vi "getSetting.vi"(7 "Array Parameter List":string[](array[string])=["izn3", "icomp"], 8 "error in (no error)":errorcluster, 9 "Parameter":string="estimator_strategy", 10 "Path":path=path "/home/ttsai/Documents/stash/ts_tcs_ofc/configData/pinv.esti", 11 "MatOper in":refnum<class "MatOper.lvclass">) -> (0 "error out":errorcluster, 2 "Value":string, 3 "MatOper out":refnum<class "MatOper.lvclass">)   [LabVIEW 2016, in "OfcFunc.lvlib" / "MatOper.lvclass"]
doc: "This vi is to read the configuration file based on the Parameter. This output can is the string. Array Parameter List defines the output with the array-like string data."
uses:
  MatOper.lvclass
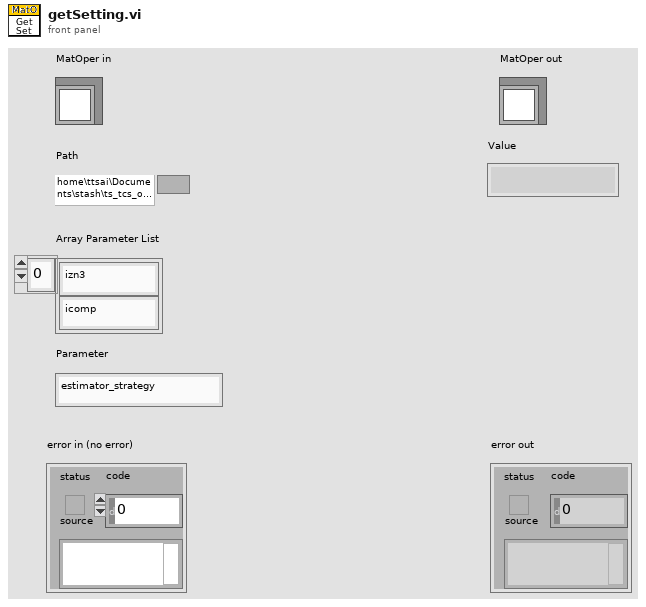
[diagram p1: front panel]
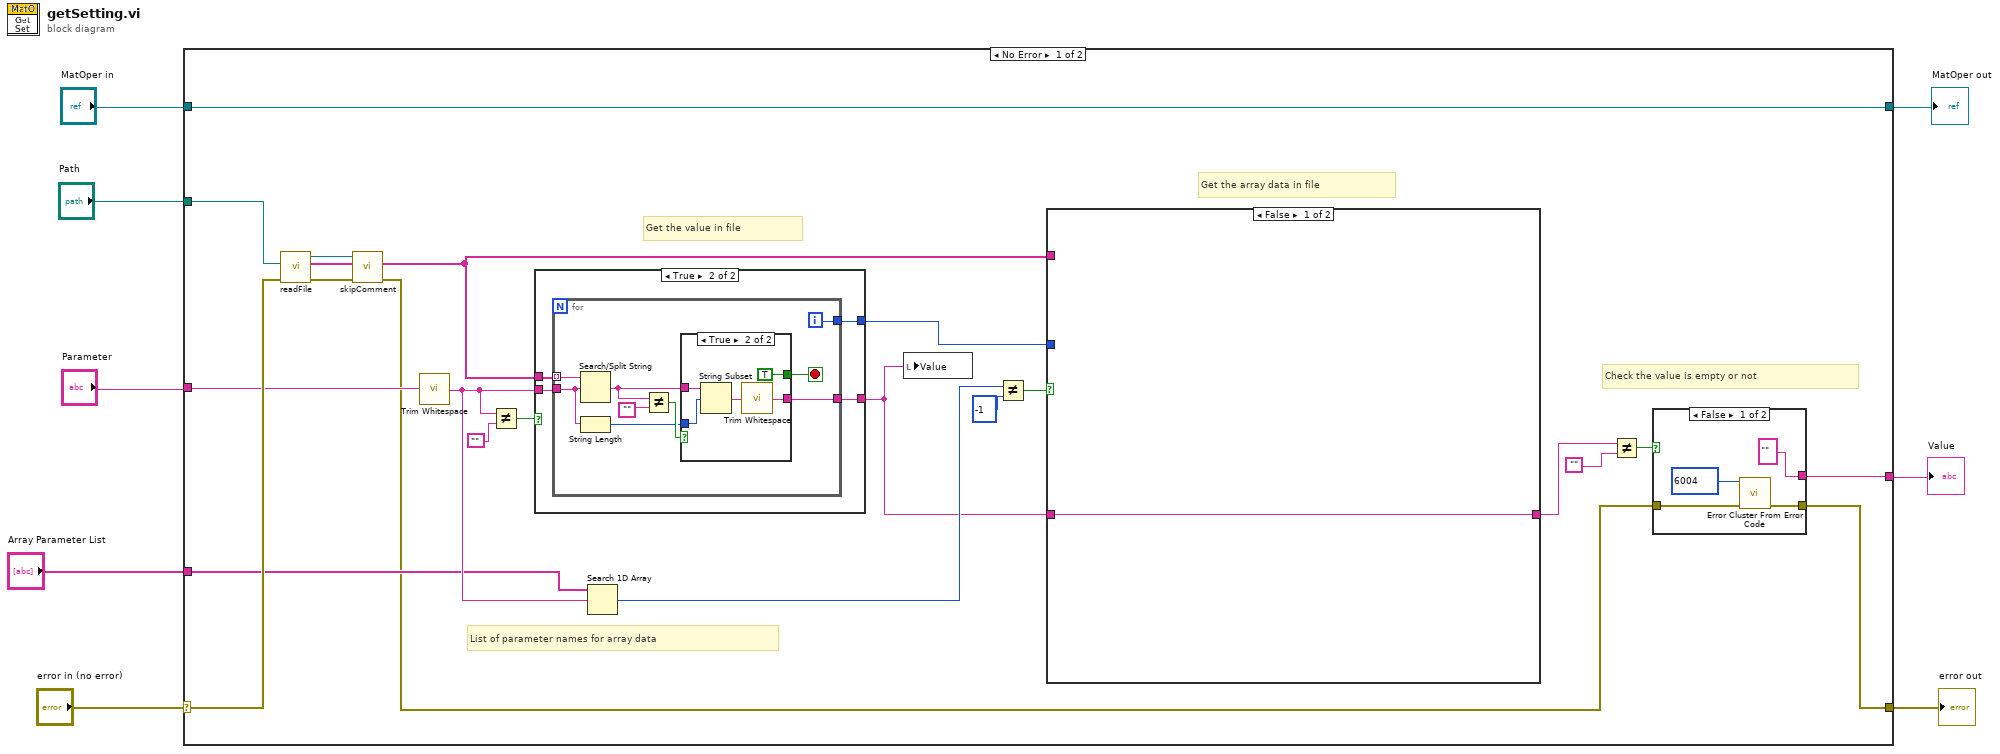
[diagram p0: block diagram]
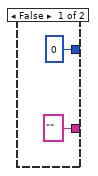
[diagram p2: hidden frame]
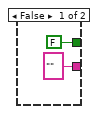
[diagram p3: hidden frame]
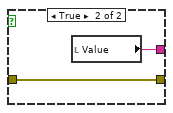
[diagram p4: hidden frame]
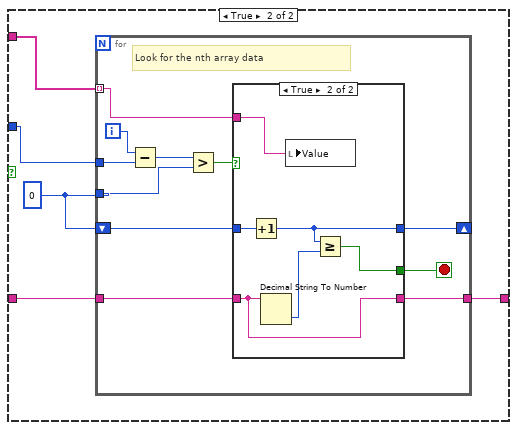
[diagram p5: hidden frame]
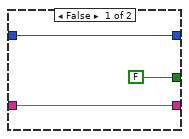
[diagram p6: hidden frame]
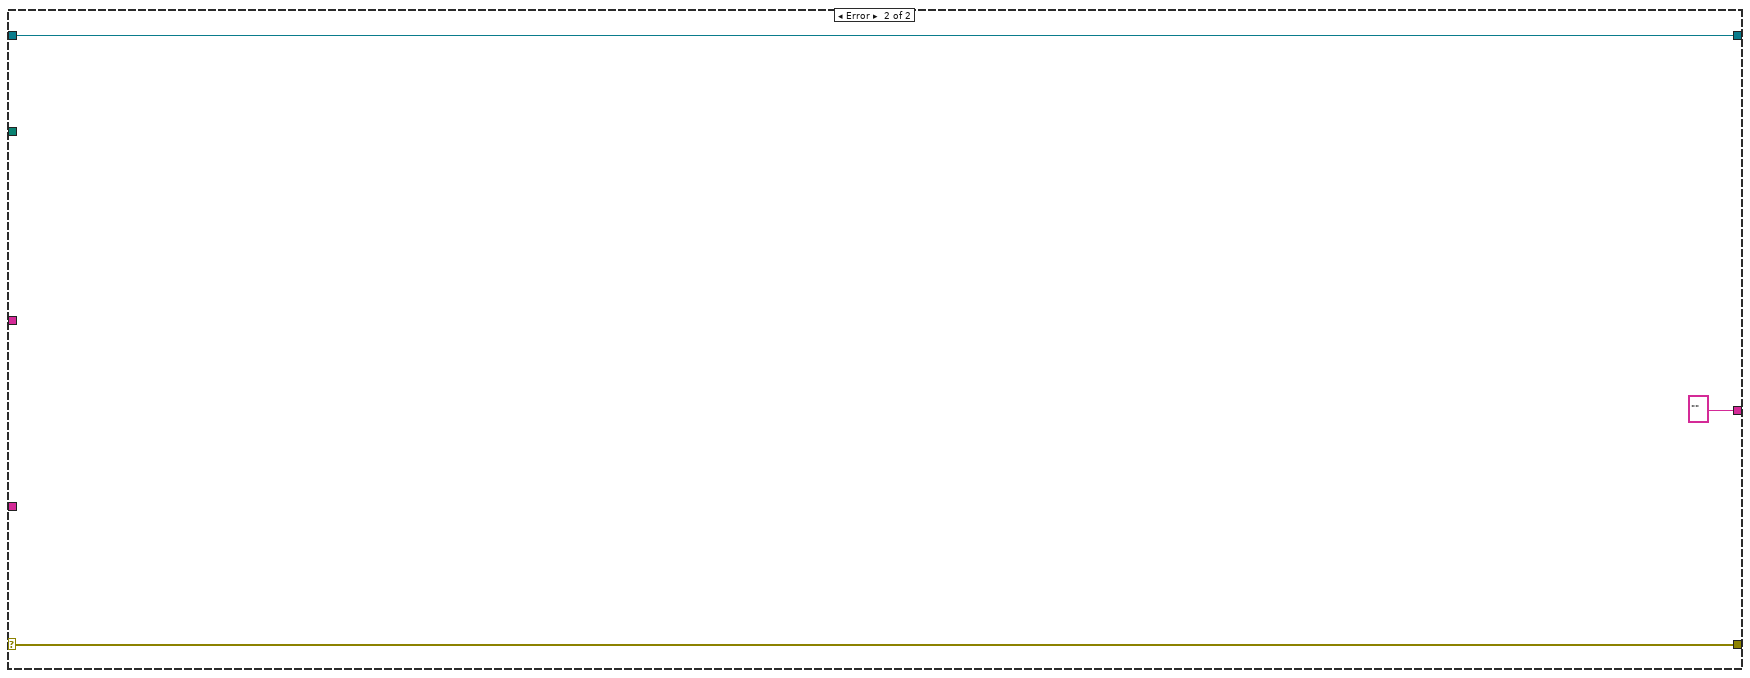
[diagram p7: hidden frame]
diagram:
  n1 = case shown="No Error" "error in (no error)" {
    selector: "error in (no error)" -> [w18 w88]
    tunnel: [w10 w88] -> w7
    tunnel: [w31 w87] -> w5
    tunnel: "MatOper in" -> [w31 w87]
    tunnel: "Path" -> [w17 _]
    tunnel: "Parameter" -> [w16 _]
    tunnel: "Array Parameter List" -> [w15 _]
    tunnel: [w9 "" ("Value")] -> w1
    frame No Error {
      # "Check the value is empty or not"
      # "List of parameter names for array data"
      # "Get the array data in file"
      # "Get the value in file"
      n2 = call "readFile.vi"("error in (no error)"=w18, "Path"=w17) -> ("error out"=w13:errorcluster, "Array"=w26:string[], "MatOper out"=w14:refnum<class "MatOper.lvclass">)  [unwired: 7 in]
      n3 = call "skipComment.vi"("error in (no error)"=w13, "Content"=w26, "MatOper in"=w14) -> ("error out"=w12:errorcluster, "Modified Content"=w25:string[])  [unwired: 6 in, 1 out]
      n4 = call <vilib>:"Trim Whitespace.vi"("string"=w16) -> ("trimmed string"=w20:string)  [unwired: 1 in]
      n5 = Not Equal?(x=w20, y="") -> (x != y?=w19:bool)
      n6 = case shown="True" w19 {
        tunnel: [0 w37] -> w27
        tunnel: ["" ("trimmed string") w36] -> w11
        tunnel: w25 -> [_ w35]
        tunnel: w20 -> [_ w34]
        frame False {
        }
        frame True {
          n7 = for {
            tunnel: w35 -> [w39] mode=indexing
            tunnel: w34 -> [w42]
            tunnel: [w41] -> w36
            tunnel: [w40] -> w37
            i -> [w40]
            stop <- w45 stop-if-true
            n8 = Search/Split String(string=w39, search string/char (-)=w42) -> (match + rest of string=w44:string)  [unwired: 1 in, 2 out]
            n9 = String Length(string=w42) -> (length=w43:i32)
            n10 = Not Equal?(x=w44, y="") -> (x != y?=w46:bool)
            n11 = case shown="True" w46 {
              tunnel: [FALSE TRUE] -> w45
              tunnel: w44 -> [_ w52]
              tunnel: ["" w49] -> w41
              tunnel: w43 -> [_ w51]
              frame False {
              }
              frame True {
                n12 = String Subset(string=w52, offset (0)=w51) -> (substring=w50:string)  [unwired: 1 in]
                n13 = call <vilib>:"Trim Whitespace.vi"("string"=w50) -> ("trimmed string"=w49:string)  [unwired: 1 in]
              }
            }
          }
        }
      }
      n14 = Search 1D Array(1D array=w15, element=w20) -> (index of element=w29:i32)  [unwired: 1 in]
      n15 = local write "Value"(w11) -> ()
      n16 = Not Equal?(x=w29, y=-1) -> (x != y?=w30:bool)
      n17 = case shown="False" w30 {
        tunnel: w27 -> [_ w65]
        tunnel: w25 -> [_ w64]
        tunnel: w11 -> [w60 w63]
        tunnel: [w60 w61] -> w22
        frame False {
        }
        frame True {
          w62 = 0 ("y")
          n18 = for {
            tunnel: w65 -> [w72]
            tunnel: w64 -> [w75] mode=indexing
            shift-right: [w68] -> _
            shift-left: w62 -> [w69]
            tunnel: w62 -> [w70]
            tunnel: w63 -> [w67]
            tunnel: [w66] -> w61
            i -> [w73]
            stop <- w71 stop-if-true
            # "Look for the nth array data"
            n19 = Subtract(x=w73, y=w72) -> (x-y=w74:i32)
            n20 = Greater?(x=w74, y=w70) -> (0:w76:bool)
            n21 = case shown="True" w76 {
              tunnel: w75 -> [_ w83]
              tunnel: [FALSE w84] -> w71
              tunnel: w69 -> [w78 w82]
              tunnel: [w78 w81] -> w68
              tunnel: w67 -> [w77 w80]
              tunnel: [w77 w80] -> w66
              frame False {
              }
              frame True {
                n22 = Increment(x=w82) -> (x+1=w81:i32)
                n23 = Decimal String To Number(string=w80) -> (number=w85:i32)  [unwired: 2 in, 1 out]
                n24 = local write "Value"(w83) -> ()
                n25 = Greater Or Equal?(x=w81, y=w85) -> (x >= y?=w84:bool)
              }
            }
          }
        }
      }
      n26 = Not Equal?(x=w22, y="") -> (x != y?=w24:bool)
      n27 = case shown="False" w24 {
        tunnel: w12 -> [w56 w59]
        tunnel: [w55 w59] -> w10
        tunnel: ["" ("Value") w58] -> w9
        frame False {
          n28 = call <vilib>:"Error Cluster From Error Code.vi"("error in (no error)"=w56, "error code (0)"=6004 ("code")) -> ("error out"=w55:errorcluster)  [unwired: 7 in]
        }
        frame True {
          n29 = local read "Value"() -> (w58:string)
        }
      }
    }
    frame Error {
    }
  }
  "error out" <- w7
  "MatOper out" <- w5
  "Value" <- w1
